vi "Blank Key Reserved String.vi"() -> (0 "Reserved characters":string)   [LabVIEW 2023, in "uLib.lvlib" / "uData.lvclass"]
doc: "Reserved ASCII string to use when a blank tag is provided. This is to prevent returning an error when handling a blank key at the private variant attributes."
uses:
  uData.lvclass
  uData.lvclass/uData.ctl
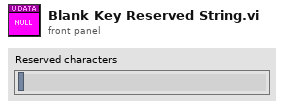
[diagram p1: front panel]
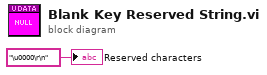
[diagram p0: block diagram]
diagram:
  "Reserved characters" <- "\u0000\r\n" ("x")
